vi "RTS Group Header.vi"(8 "error in (no error)":errorcluster, 11 "Refnum in":refnum<k34>) -> (0 "error out":errorcluster, 1 "group names":string[](array[string]), 2 "group/channel names":string[](array[string]), 3 "Refnum out":refnum<k34>)   [LabVIEW 2016]
panel:
  out "group/channel names 2":string[][](array[string])
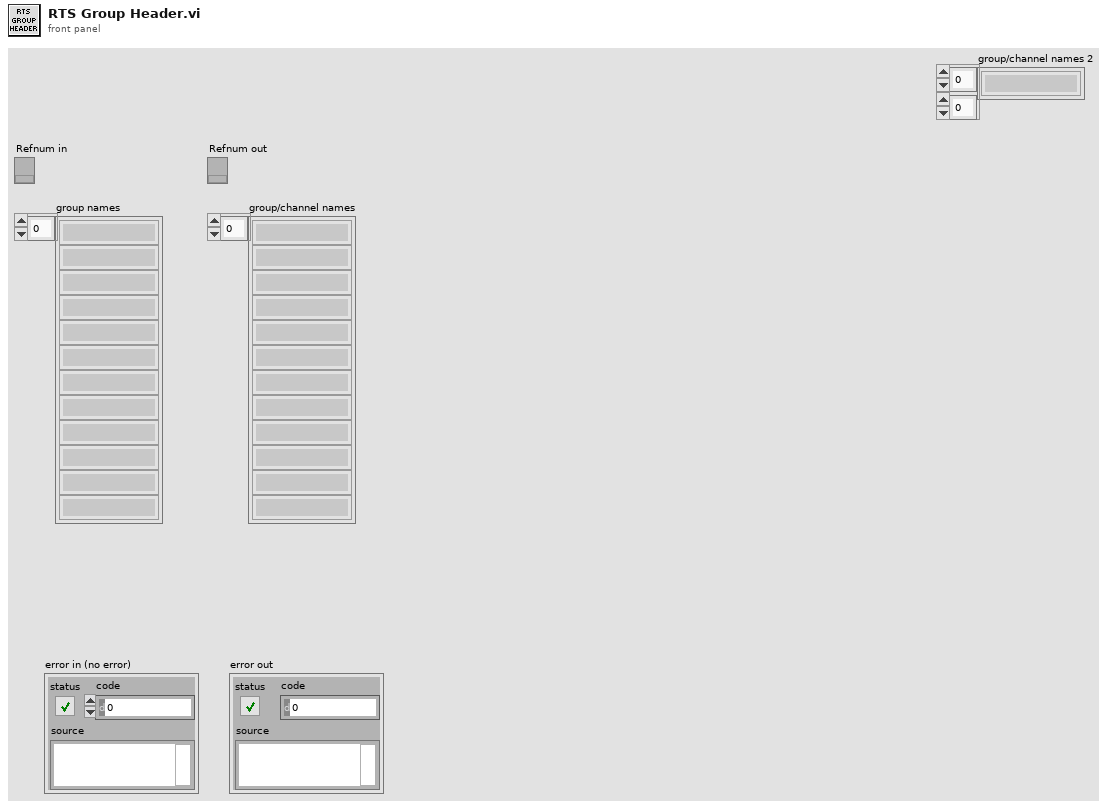
[diagram p1: front panel]
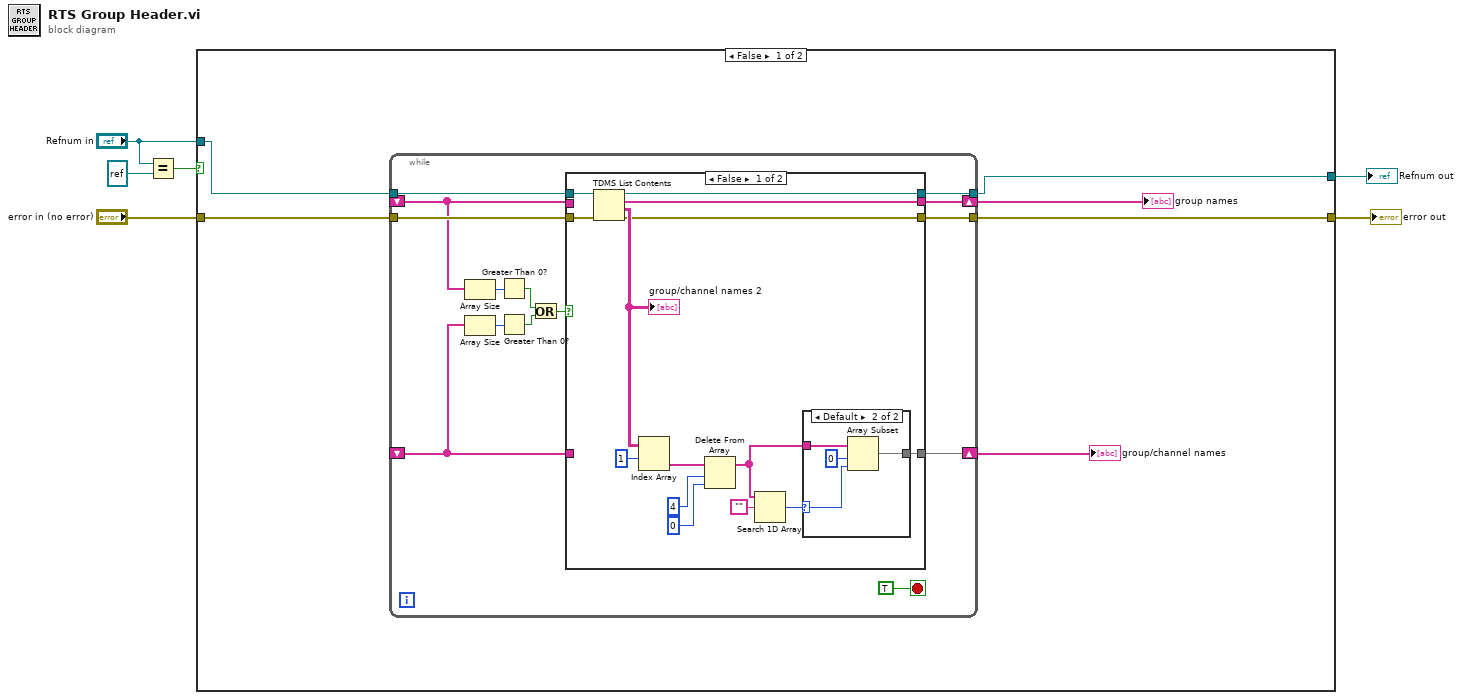
[diagram p0: block diagram]
diagram:
  n1 = Equal?(x="Refnum in", y=refnum<k34> refnum ("TDMS File 8")) -> (x = y?=w2:bool)
  n2 = case shown="False" w2 {
    tunnel: "Refnum in" -> [w12 w50]
    tunnel: [w9 w51] -> w6
    tunnel: "error in (no error)" -> [w8 w51]
    tunnel: [w7 w50] -> w1
    frame False {
      n3 = while {
        shift-right: [w21] -> w10
        shift-left: _ -> [w13]
        shift-right: [w22] -> w11
        shift-left: _ -> [w17]
        tunnel: w12 -> [w24]
        tunnel: [w23] -> w7
        tunnel: w8 -> [w26]
        tunnel: [w25] -> w9
        stop <- TRUE stop-if-true
        n4 = Array Size(array=w13) -> (size(s)=w19:i32)
        n5 = Array Size(array=w17) -> (size(s)=w18:i32)
        n6 = Greater Than 0?(x=w19) -> (x > 0?=w16:bool)
        n7 = Greater Than 0?(x=w18) -> (x > 0?=w15:bool)
        n8 = Or(x=w16, y=w15) -> (x .or. y?=w14:bool)
        n9 = case shown="False" w14 {
          tunnel: w26 -> [w36 w48]
          tunnel: [w35 w48] -> w25
          tunnel: w24 -> [w34 w49]
          tunnel: [w33 w49] -> w23
          tunnel: [w29 w46] -> w22
          tunnel: [w32 w47] -> w21
          tunnel: w13 -> [_ w47]
          tunnel: w17 -> [_ w46]
          frame False {
            n10 = TDMS List Contents(4:w36, 7:w34) -> (0:w35:errorcluster, 1:w39:string[][], 2:w32:string[], 3:w33:refnum<k34>)  [unwired: 1 in]
            "group/channel names 2" <- w39
            n11 = Index Array(array=w39, index (row)=1 ("disabled index (col)")) -> (element=w31:string[])  [unwired: 1 in]
            n12 = Delete From Array(array=w31, length=4, index=0) -> (array with subset deleted=w30:string[])  [unwired: 1 out]
            n13 = Search 1D Array(1D array=w30, element="") -> (index of element=w28:i32)  [unwired: 1 in]
            n14 = case shown="Default" w28 {
              selector: w28 -> [_ w42]
              tunnel: w30 -> [w41 w44]
              tunnel: [w41 w43] -> w29
              frame -1 {
              }
              frame Default {
                n15 = Array Subset(array=w44, index=0, length=w42) -> (w43:string[])
              }
            }
          }
          frame True {
          }
        }
      }
      "group/channel names" <- w11
      "group names" <- w10
    }
    frame True {
    }
  }
  "error out" <- w6
  "Refnum out" <- w1
